vi "waypoint_icon_to_bitmap.vi"(8 "Index":i32, 9 "Done?":bool, 10 "Mission Waypoint?":bool, 11 "Waypoint Icon References":T1) -> (1 "Icon Bitmap Out":u32[][](array[colorbox]), 3 "Icon Out":T2(plugin-control))   [LabVIEW 2013]
doc: "Rotates icon images of the boat and sails and overlays them on each other to create a representation of the current state of the robot. Also converts the output image to a bitmap for easy overlay on the mission map.\n\norigininally by Jason Curtis\nAdapted 4/5/2014 by Mac-I Crowell"
uses:
  TypeDef/waypoint_icon_references.ctl
  <vilib>/vision/Image Controls.llb/IMAQ Image.ctl
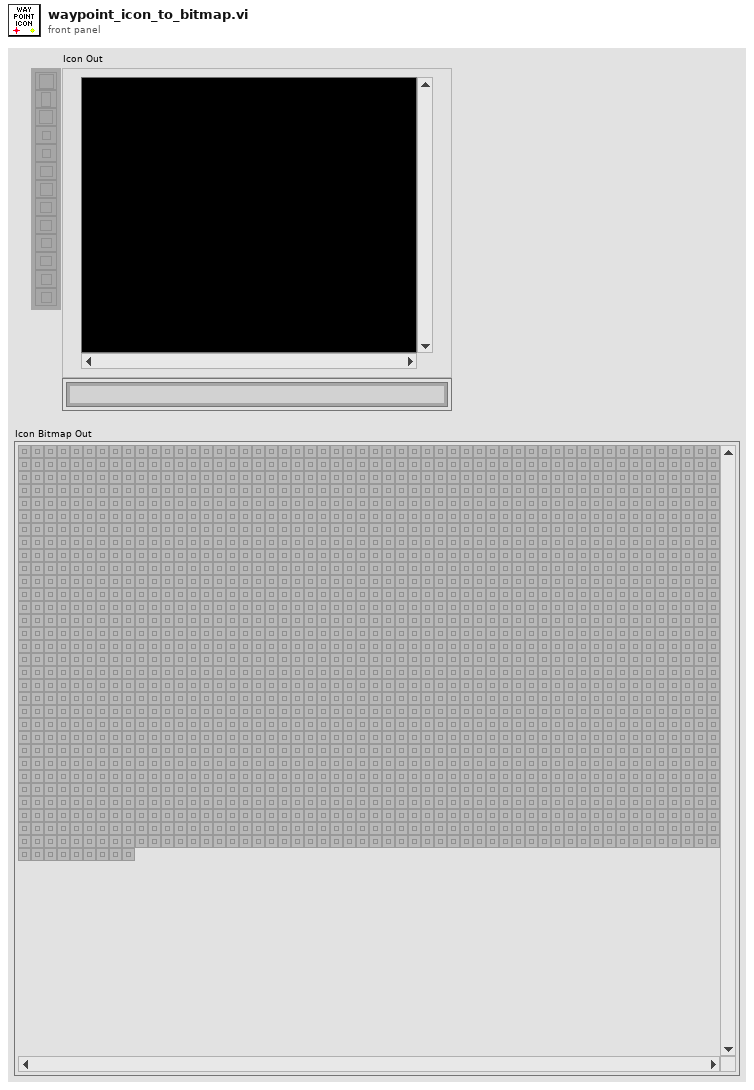
[diagram p1: front panel]
types:
  T1 = typedef "waypoint_icon_references.ctl" = cluster{"Mission Waypoint Icon":T2, "Sailing Point Icon":T2, "Mission Waypoint Done Icon":T2, "Sailing Point Done Icon":T2, "Next Mission Waypoint Icon":T2, "Next Sailing Point Icon":T2}
  T2 = typedef "IMAQ Image.ctl" = refnum<image>
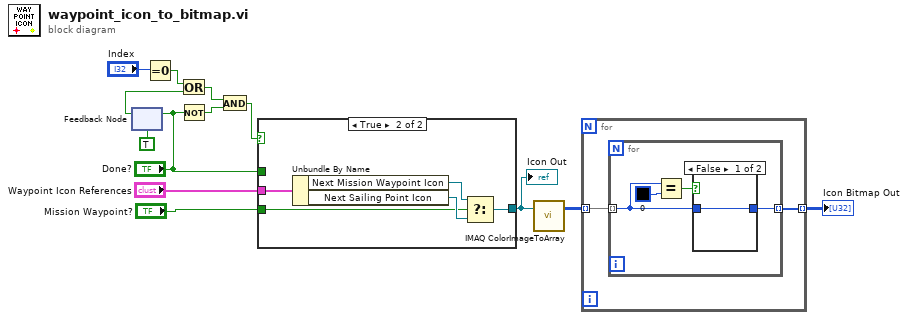
[diagram p0: block diagram]
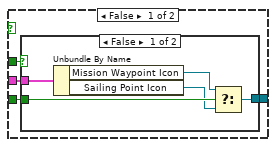
[diagram p2: hidden frame]
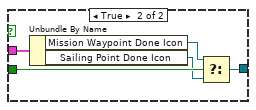
[diagram p3: hidden frame]
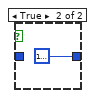
[diagram p4: hidden frame]
diagram:
  n1 = feedback-in #1("Done?") -> ()
  n2 = feedback #1(TRUE ("Done?")) -> (w4:bool)
  n3 = Equal To 0?(x="Index") -> (x = 0?=w3:bool)
  n4 = Or(x=w3, y=w4) -> (x .or. y?=w5:bool)
  n5 = Not(x="Done?") -> (.not. x?=w8:bool)
  n6 = And(x=w5, y=w8) -> (x .and. y?=w1:bool)
  n7 = case shown="True" w1 {
    tunnel: "Waypoint Icon References" -> [w17 w28]
    tunnel: "Mission Waypoint?" -> [w16 w29]
    tunnel: [w15 w31] -> w9
    tunnel: "Done?" -> [w14 _]
    frame False {
      n8 = case shown="False" w14 {
        tunnel: w17 -> [w21 w27]
        tunnel: w16 -> [w22 w26]
        tunnel: [w18 w23] -> w15
        frame False {
          n9 = Unbundle By Name(w21) -> ("Mission Waypoint Icon"=w20:T2, "Sailing Point Icon"=w19:T2)
          n10 = Select(t=w20, s=w22, f=w19) -> (s? t:f=w18:T2)
        }
        frame True {
          n11 = Unbundle By Name(w27) -> ("Mission Waypoint Done Icon"=w25:T2, "Sailing Point Done Icon"=w24:T2)
          n12 = Select(t=w25, s=w26, f=w24) -> (s? t:f=w23:T2)
        }
      }
    }
    frame True {
      n13 = Unbundle By Name(w28) -> ("Next Mission Waypoint Icon"=w32:T2, "Next Sailing Point Icon"=w30:T2)
      n14 = Select(t=w32, s=w29, f=w30) -> (s? t:f=w31:T2)
    }
  }
  "Icon Out" <- w9
  n15 = call "IMAQ ColorImageToArray"("Image"=w9) -> ("Image Pixels (U32)"=w12:u32[][])  [unwired: 2 in, 3 out]
  n16 = for {
    tunnel: w12 -> [w34] mode=indexing
    tunnel: [w33] -> w13 mode=indexing
    n17 = for {
      tunnel: w34 -> [w36] mode=indexing
      tunnel: [w37] -> w33 mode=indexing
      n18 = Equal?(x=w36, y=u32 0) -> (x = y?=w38:bool)
      n19 = case shown="False" w38 {
        tunnel: [w39 u32 16777216] -> w37
        tunnel: w36 -> [w39 _]
        frame False {
        }
        frame True {
        }
      }
    }
  }
  "Icon Bitmap Out" <- w13
